vi "Plot Zoom.vi"(7 "Control Ref Queue":T1, 8 "error in (no error)":errorcluster, 9 "Zoom Mode":bool, 11 "3D Plot.lvclass in":refnum<class "3D Plot.lvclass">) -> (0 "error out":errorcluster, 1 "Dup Ortho Zoom Mode":bool, 3 "3D Plot.lvclass out":refnum<class "3D Plot.lvclass">, 4 "View Distance Out":sgl)   [LabVIEW 2020, in "3D Plot.lvclass"]
uses:
  3D Plot.lvclass
  3DMathPlot Ctrl Act Queue.ctl
  3DMathPlot Ctrl Act Cluster.ctl
  3DMathPlot State Class.ctl
  3D Plot.lvclass/3D Plot.ctl
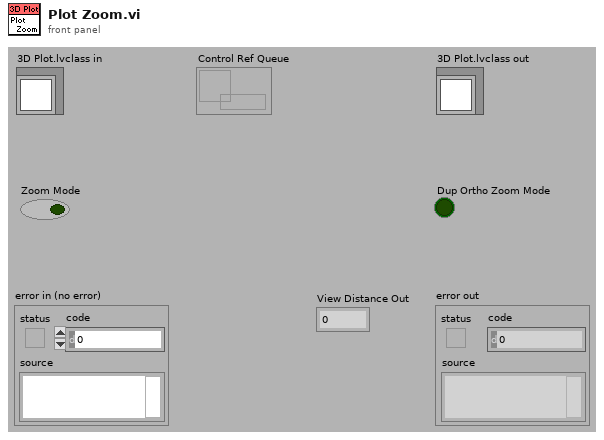
[diagram p1: front panel]
types:
  T1 = typedef "3DMathPlot Ctrl Act Queue.ctl" = refnum<queue>
  T2 = typedef "3DMathPlot Ctrl Act Cluster.ctl" = cluster{"3D Picture Control":refnum<vi>, "Render Window Refnum":refnum<vi>, "XY Graph":refnum<vi>, "Intensity Graph":refnum<vi>, "Color Legend Palette":refnum<vi>, "Projection Palette":refnum<vi>, "XControl  Ref":refnum<vi>, "Facade Ref":refnum<vi>, "Export Image Ref":refnum<vi>, "Clear Data Flag":bool, "Display State Change Class":T3}
  T3 = typedef "3DMathPlot State Class.ctl" = enum16{"Update All Objects (Undo)", "Update Light Object Only", "Update Axis Object Only", "Update Plot Object Only", "Update Cursor Object Only", "Update Axis Plot Cursor Objects", "No Update"}
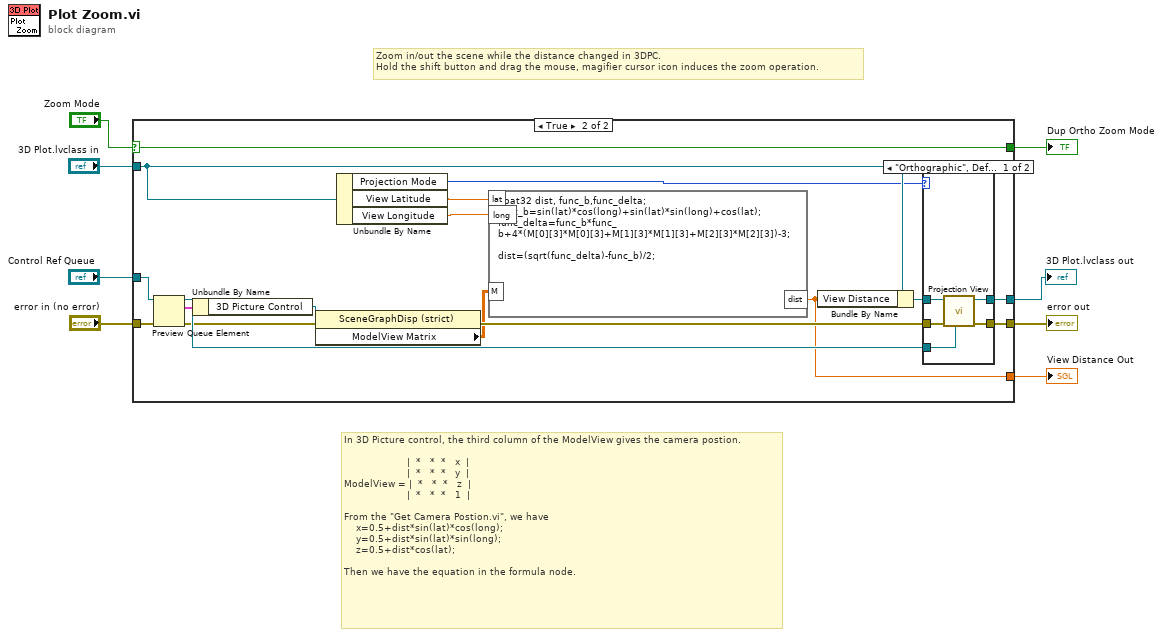
[diagram p0: block diagram]
diagram:
  # "Zoom in/out the scene while the distance changed in 3DPC.\nHold the shift button and drag the mouse, magifier cursor icon induces the zoom operation."
  # "In 3D Picture control, the third column of the ModelView gives the camera postion.\n\n                     |  *   *  *   x  |\n                     |  *   *  *   y  |\nModelView = |  *   *  *   z  |\n                     |  *   *  *   1  |\n\nFrom the \"Get Camera Postion.vi\", we have\n    x=0.5+dist*sin(lat)*cos(long);\n    y=0.5+dist*sin(lat)*sin(long);\n    z=0.5+dist*cos(lat);\n\nThen we have the equation in the formula node."
  n1 = case shown="True" "Zoom Mode" {
    selector: "Zoom Mode" -> [w11 w28]
    tunnel: [w11 w28] -> w8
    tunnel: "3D Plot.lvclass in" -> [w10 w27]
    tunnel: [w10 w25] -> w2
    tunnel: [_ w13] -> w1
    tunnel: "error in (no error)" -> [w9 w20]
    tunnel: [w9 w24] -> w6
    tunnel: "Control Ref Queue" -> [_ w23]
    frame False {
    }
    frame True {
      n2 = Preview Queue Element(queue=w23, error in (no error)=w20) -> (queue out=w18:T1, element=w22:T2, error out=w17:errorcluster)  [unwired: 2 out]
      n3 = Unbundle By Name(w22) -> ("3D Picture Control"=w19:refnum<vi>)
      n4 = property class="SceneGraphDisp (strict)"(reference=w19, error in=w17) -> (error out=w16:errorcluster, "ModelView Matrix"=w12:sgl[][])  [unwired: 1 out]
      n5 = Unbundle By Name(w27) -> ("Projection Mode"=w21:enum16{"Orthographic", "Perspective"}, "View Latitude"=w15:sgl, "View Longitude"=w14:sgl)
      n6 = formula code="float32 dist, func_b,func_delta;\nfunc_b=sin(lat)*cos(long)+sin(lat)*sin(long)+cos(lat);\nfunc_delta=func_b*func_b+4*(M[0][3]*M[0][3]+M[1][3]*M[1][3]+M[2][3]*M[2][3])-3;\n\ndist=(sqrt(func_delta)-func_b)/2;"("M"=w12, "lat"=w15, "long"=w14) -> ("dist"=w13:sgl)
      n7 = Bundle By Name(cluster=w27, "View Distance"=w13) -> (w26:refnum<class "3D Plot.lvclass">)
      n8 = case shown="\"Orthographic\", Default" w21 {
        tunnel: w26 -> [w33 w35]
        tunnel: [w32 w35] -> w25
        tunnel: w16 -> [w31 w34]
        tunnel: [w30 w34] -> w24
        tunnel: w18 -> [w29 _]
        frame "Orthographic", Default {
          n9 = call "Projection View.vi"("Control Ref Queue"=w29, "error in (no error)"=w31, "3D Plot.lvclass in"=w33) -> ("error out"=w30:errorcluster, "3D Plot.lvclass out"=w32:refnum<class "3D Plot.lvclass">)  [unwired: 1 in, 6 out]
        }
        frame "Perspective" {
        }
      }
    }
  }
  "Dup Ortho Zoom Mode" <- w8
  "error out" <- w6
  "3D Plot.lvclass out" <- w2
  "View Distance Out" <- w1
